vi "getRect.vi"(8 "error in (no error)":errorcluster, 11 "GObject in":refnum<class "GObject.lvclass">) -> (0 "error out":errorcluster, 2 "rectangle":T1, 3 "GObject out":refnum<class "GObject.lvclass">)   [LabVIEW 2023, in "TLC_Scripto.lvlib" / "GObject.lvclass"]
uses:
  GObject.lvclass
  Ctrls/rectangle.ctl
  Read ref.vi
  GObject.lvclass/GObject.ctl
  TLC_Scripto.lvlib
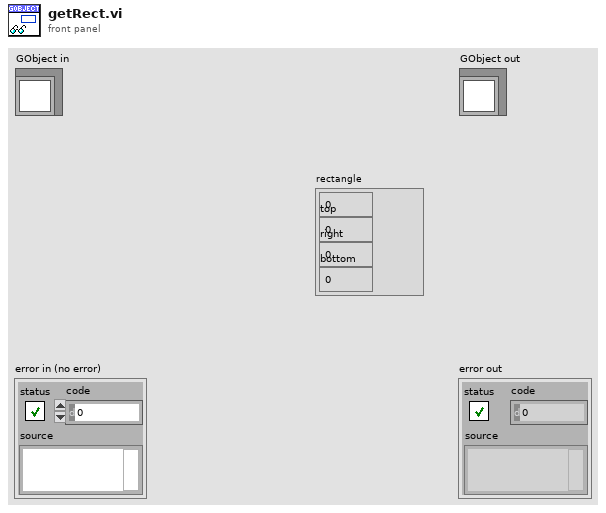
[diagram p1: front panel]
types:
  T1 = typedef "TLC_Scripto.lvlib/rectangle.ctl" = cluster{"left":i32, "top":i32, "right":i32, "bottom":i32}
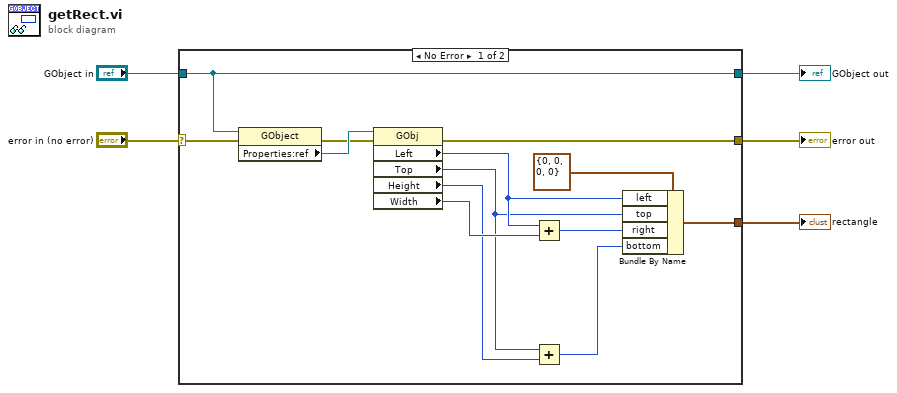
[diagram p0: block diagram]
diagram:
  n1 = case shown="No Error" "error in (no error)" {
    selector: "error in (no error)" -> [w11 w20]
    tunnel: [w10 w20] -> w4
    tunnel: [w18 w19] -> w2
    tunnel: "GObject in" -> [w18 w19]
    tunnel: [w13 _] -> w1
    frame No Error {
      n2 = property class="GObject"(reference=w18, error in=w11) -> (error out=w12:errorcluster, "Properties:ref"=w17:refnum<vi>)  [unwired: 1 out]
      n3 = property class="GObj"(reference=w17, error in=w12) -> (error out=w10:errorcluster, "Left"=w9:i32, "Top"=w8:i32, "Height"=w14:u32, "Width"=w15:u32)  [unwired: 1 out]
      n4 = Add(x=w9, y=w15) -> (x+y=w6:u32)
      n5 = Add(x=w8, y=w14) -> (x+y=w7:u32)
      n6 = Bundle By Name(cluster=T1 {"left"=0, "top"=0, "right"=0, "bottom"=0} ("rectangle"), "left"=w9, "top"=w8, "right"=w6, "bottom"=w7) -> (w13:T1)
    }
    frame Error {
    }
  }
  "error out" <- w4
  "GObject out" <- w2
  "rectangle" <- w1
